vi "Update and Check Threshold Timers.vi"(0 "[Prev Threshold Timers]":T3(array[cluster]), 1 "Current Tick Count":u32, 2 "[Threshold Settings]":string[][](array[string]), 3 "[Threshold Settings Present Bools]":bool[][](array[boolean]), 4 "[Parsed Controls]":T1, 5 "error in (no error)":errorcluster, 7 "Current RPM":dbl) -> (14 "[New Threshold Timers]":T3(array[cluster]), 16 "[Alerts] out":T4[](array[typedef]), 19 "error out":errorcluster)   [LabVIEW 2018, in "RT - Analysis.lvlib"]
uses:
  RT - Analysis.lvlib
  Public Controls/Alert Data.ctl
  Private Controls/Parsed Data Arrays.ctl
  Top Level/Shared Controls/Parsed Tag Cluster.ctl
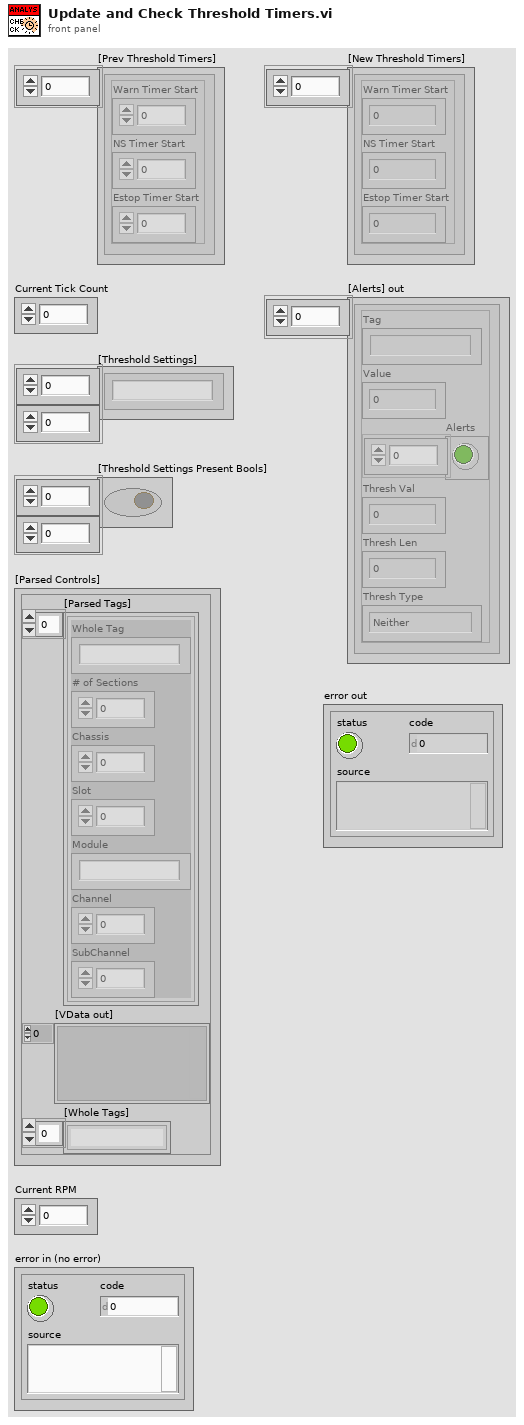
[diagram p1: front panel]
types:
  T1 = typedef "RT - Analysis.lvlib/Parsed Data Arrays.ctl" = cluster{"[Parsed Tags]":T2[], "[VData out]":variant[], "[Whole Tags]":string[]}
  T2 = typedef "Parsed Tag Cluster.ctl" = cluster{"Whole Tag":string, "# of Sections":u8, "Chassis":u8, "Slot":u8, "Module":string, "Channel":u8, "SubChannel":u8}
  T3 = cluster{"Warn Timer Start":u32, "NS Timer Start":u32, "Estop Timer Start":u32}[]
  T4 = typedef "RT - Analysis.lvlib/Alert Data.ctl" = cluster{"Tag":string, "Value":dbl, "Alerts":bool[], "Thresh Val":dbl, "Thresh Len":dbl, "Thresh Type":enum16{"Neither", "Max", "Min"}}
  T5 = cluster{"Warn Timer Start":u32, "NS Timer Start":u32, "Estop Timer Start":u32}
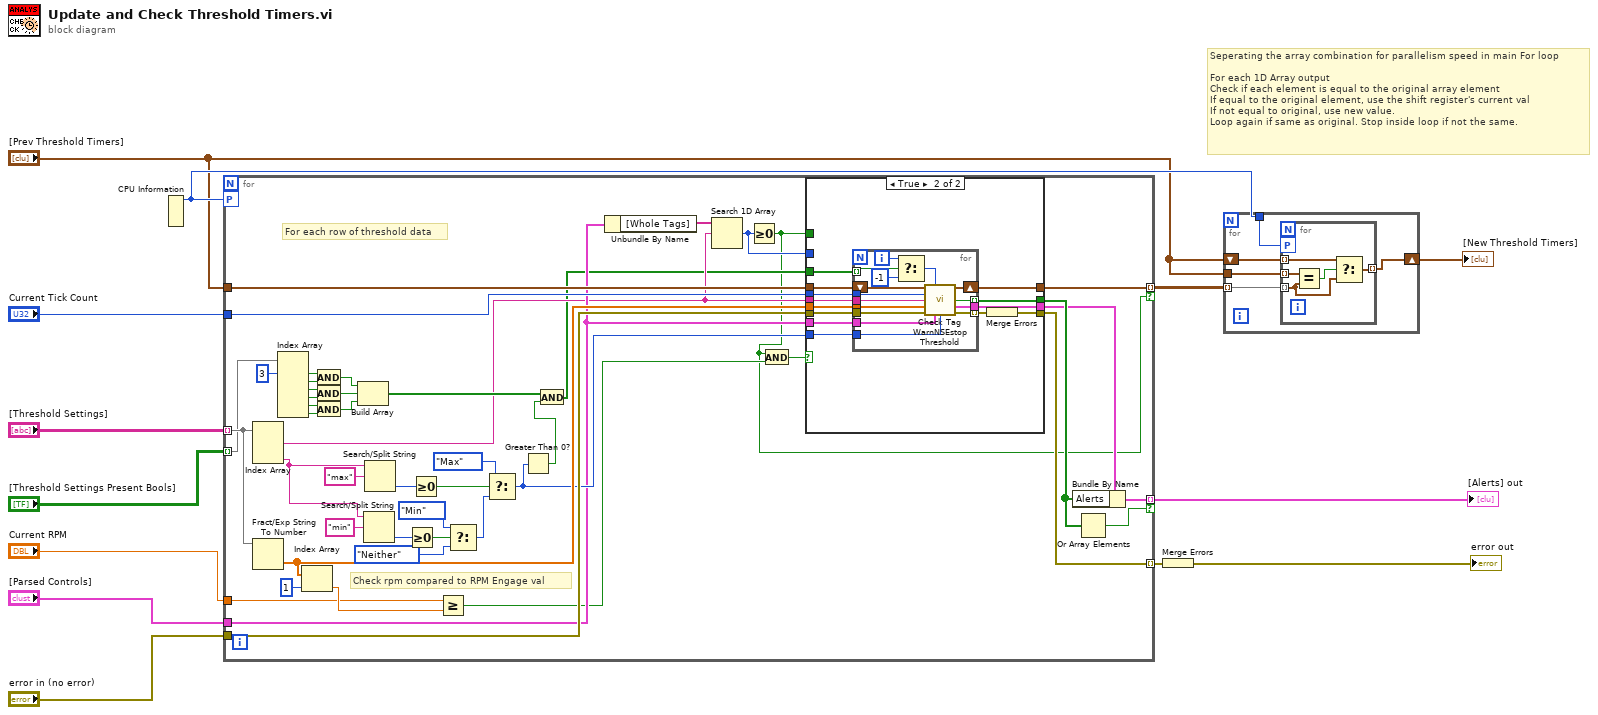
[diagram p0: block diagram]
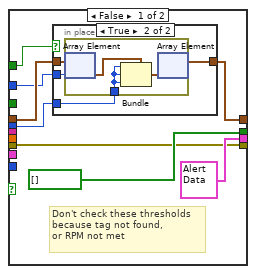
[diagram p2: hidden frame]
diagram:
  # "Seperating the array combination for parallelism speed in main For loop\n\nFor each 1D Array output\nCheck if each element is equal to the original array element\nIf equal to the original element, use the shift register's current val\nIf not equal to original, use new value.\nLoop again if same as original. Stop inside loop if not the same."
  n1 = CPU Information() -> (4:w12:i32)  [unwired: 3 out]
  n2 = for {
    tunnel: "[Threshold Settings]" -> [w60] mode=indexing
    tunnel: "error in (no error)" -> [w59]
    tunnel: [w58] -> w2 mode=indexing
    tunnel: "[Parsed Controls]" -> [w20]
    tunnel: "[Prev Threshold Timers]" -> [w57]
    tunnel: [w54] -> w5 mode=indexing if=w14
    tunnel: "Current Tick Count" -> [w56]
    tunnel: "[Threshold Settings Present Bools]" -> [w47] mode=indexing
    tunnel: [w31] -> w11 mode=indexing if=w32
    tunnel: "Current RPM" -> [w25]
    workers-P: w12 -> [_]
    # "Check rpm compared to RPM Engage val"
    # "For each row of threshold data"
    n3 = Index Array(array=w60) -> (element #1=w19:string, element #3=w30:string)  [unwired: 3 in, 1 out]
    n4 = Fract/Exp String To Number(string=w60) -> (number=w29:dbl[])  [unwired: 3 in, 1 out]
    n5 = Index Array(array=w47, index #1=3 ("index")) -> (element #1=w48:bool, element #2=w49:bool, element #3=w50:bool, element #4=w53:bool, element #5=w51:bool, element #6=w52:bool)  [unwired: 5 in]
    n6 = Index Array(array=w29, index=1) -> (element=w26:dbl)
    n7 = And(x=w48, y=w49) -> (x .and. y?=w45:bool)
    n8 = And(x=w50, y=w53) -> (x .and. y?=w46:bool)
    n9 = And(x=w51, y=w52) -> (x .and. y?=w44:bool)
    n10 = Build Array(w45, w46, w44) -> (w55:bool[])
    n11 = Search/Split String(string=w30, search string/char (-)="min") -> (offset of match=w39:i32)  [unwired: 1 in, 2 out]
    n12 = Search/Split String(string=w30, search string/char (-)="max") -> (offset of match=w42:i32)  [unwired: 1 in, 2 out]
    n13 = Greater Or Equal To 0?(x=w39) -> (x >= 0?=w34:bool)
    n14 = Greater Or Equal To 0?(x=w42) -> (x >= 0?=w35:bool)
    n15 = Greater Or Equal?(x=w25, y=w26) -> (x >= y?=w17:bool)
    n16 = Select(t=enum16{"Neither", "Max", "Min"}."Min", s=w34, f=enum16{"Neither", "Max", "Min"}."Neither") -> (s? t:f=w38:enum16{"Neither", "Max", "Min"})
    n17 = Select(t=enum16{"Neither", "Max", "Min"}."Max", s=w35, f=w38) -> (s? t:f=w28:enum16{"Neither", "Max", "Min"})
    n18 = Greater Than 0?(x=w28) -> (x > 0?=w33:bool)
    n19 = And(x=w55, y=w33) -> (x .and. y?=w15:bool[])
    n20 = Unbundle By Name(w20) -> ("[Whole Tags]"=w21:string[])
    n21 = Search 1D Array(1D array=w21, element=w19) -> (index of element=w16:i32)  [unwired: 1 in]
    n22 = Greater Or Equal To 0?(x=w16) -> (x >= 0?=w14:bool)
    n23 = And(x=w14, y=w17) -> (x .and. y?=w18:bool)
    n24 = case shown="True" w18 {
      tunnel: w59 -> [w66 w89]
      tunnel: [w66 w88] -> w58
      tunnel: w20 -> [_ w87]
      tunnel: w57 -> [w65 w86]
      tunnel: w56 -> [w62 w85]
      tunnel: [w64 w84] -> w54
      tunnel: w15 -> [_ w77]
      tunnel: w19 -> [_ w83]
      tunnel: w29 -> [_ w82]
      tunnel: w28 -> [_ w81]
      tunnel: [bool[] [] w80] -> w24
      tunnel: [T4 {"Tag"="", "Value"=0.0, "Alerts"=[], "Thresh Val"=0.0, "Thresh Len"=0.0, "Thresh Type"=enum."Neither"} ("Tag Thresh Info") w79] -> w23
      tunnel: w16 -> [w63 _]
      tunnel: w14 -> [w61 _]
      frame False {
        # "Don't check these thresholds\nbecause tag not found,\nor RPM not met"
        n25 = case shown="True" w61 {
          tunnel: w65 -> [w69 w73]
          tunnel: [w69 w72] -> w64
          tunnel: w63 -> [_ w71]
          tunnel: w62 -> [_ w70]
          frame False {
          }
          frame True {
            n26 = in-place {
              in-place-border: w70 -> [w74]
              n27 = in-place-array #1(w73, w71) -> (w76:T5)
              n28 = Bundle(cluster=w76, "Warn Timer Start"=w74, "NS Timer Start"=w74, "Estop Timer Start"=w74) -> (w75:T5)
              n29 = in-place-array #1(w75) -> (w72:T3)  [unwired: 1 out]
            }
          }
        }
      }
      frame True {
        n30 = for {
          tunnel: w85 -> [w101]
          tunnel: w82 -> [w100]
          tunnel: w83 -> [w99]
          tunnel: w87 -> [w98]
          tunnel: w89 -> [w104]
          tunnel: [w103] -> w78 mode=indexing
          tunnel: w77 -> [w95] mode=indexing
          shift-right: [w102] -> w84
          shift-left: w86 -> [w97]
          tunnel: [w92] -> w80 mode=indexing
          tunnel: w81 -> [w91]
          tunnel: [w90] -> w79
          i -> [w94]
          n31 = Select(t=w94, s=w95, f=-1) -> (s? t:f=w96:i32)
          n32 = call "Check Tag WarnNSEstop Threshold.vi"("Tick Counts Since Last Over Threshold"=w97, "Warn/NS/Estop (0/1/2)"=w96, "Current Tick Count"=w101, "Tag from APU Setup File"=w99, "Row of Tag/Warn/NS/Estop Vals"=w100, "error in (no error)"=w104, "Parsed Tags in"=w98, "Threshold Type (Neither/Max/Min)"=w91) -> ("Tick Counts Since Last Over Threshold out"=w102:T3, "Alert"=w92:bool, "Tag Thresh Info"=w90:T4, "error out"=w103:errorcluster)  [unwired: 4 in]
        }
        n33 = Merge Errors(w78) -> (w88:errorcluster)
      }
    }
    n34 = Bundle By Name(cluster=w23, "Alerts"=w24) -> (w31:T4)
    n35 = Or Array Elements(Boolean array=w24) -> (logical OR=w32:bool)
  }
  "[Alerts] out" <- w11
  n36 = Merge Errors(w2) -> (→"error out":errorcluster)
  n37 = for {
    tunnel: w5 -> [w109] mode=indexing
    shift-right: [w108] -> w7
    shift-left: "[Prev Threshold Timers]" -> [w107]
    tunnel: "[Prev Threshold Timers]" -> [w106]
    tunnel: w12 -> [w105]
    n38 = for {
      tunnel: w109 -> [w112] mode=indexing
      tunnel: [w114] -> w108 mode=indexing
      tunnel: w107 -> [w111] mode=indexing
      tunnel: w106 -> [w113] mode=indexing
      workers-P: w105 -> [_]
      n39 = Equal?(x=w113, y=w112) -> (x = y?=w110:bool)
      n40 = Select(t=w111, s=w110, f=w112) -> (s? t:f=w114:T5)
    }
  }
  "[New Threshold Timers]" <- w7
